vi "rmad mesh to file.vi"(0 "Mote Status":T1(array[cluster]) {"mote state" items=["Lost"=0, "Negotiating"=1, "Operational"=4]}, 3 "mesh datadir":string, 5 "Primary link status":T3(array[cluster]), 9 "last packet type dust":i32[](array[numeric]), 11 "error in":errorcluster, 13 "mac adresses":T2) -> (15 "error out":errorcluster)   [LabVIEW 2017]
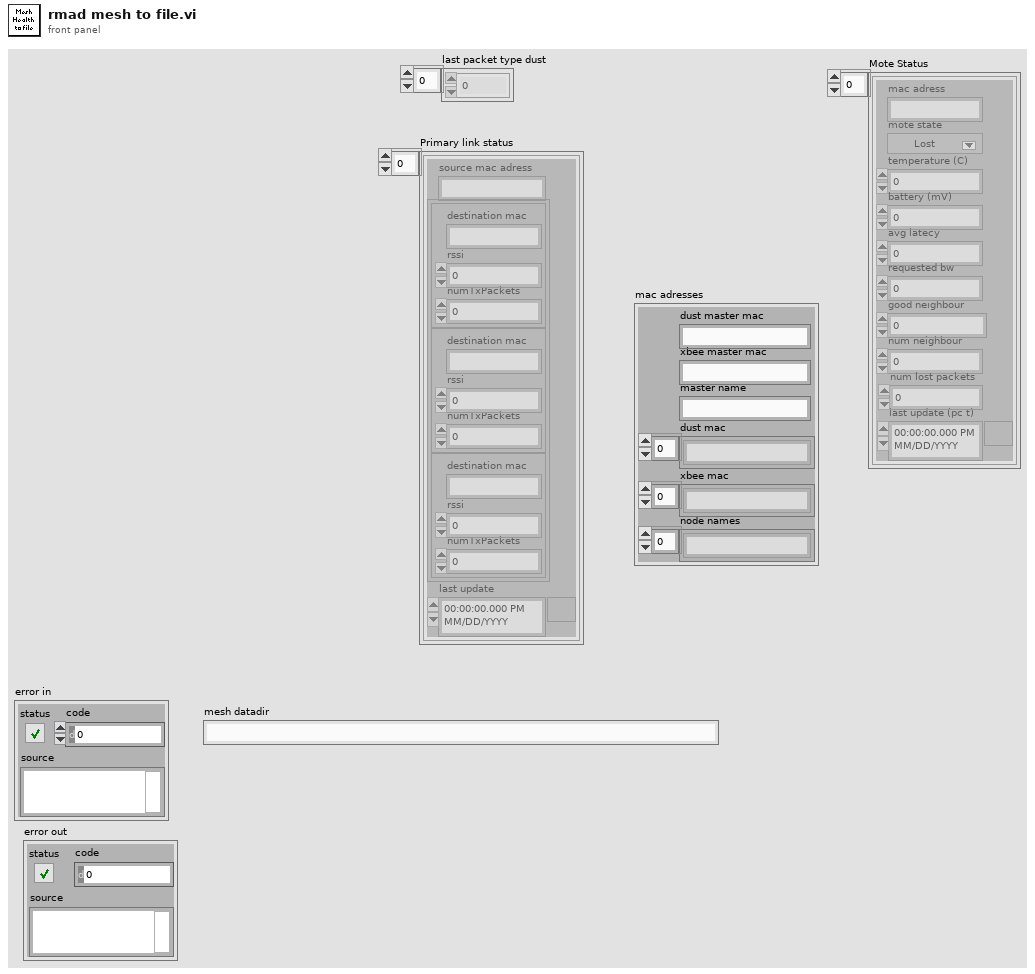
[diagram p1: front panel]
types:
  T1 = cluster{"mac adress":string, "mote state":u8, "temperature (C)":i8, "battery (mV)":u16, "avg latecy":u32, "requested bw":u32, "good neighbour":u8, "num neighbour":u8, "num lost packets":u8, "last update (pc t)":timestamp}[]
  T2 = cluster{"dust master mac":string, "xbee master mac":string, "master name":string, "dust mac":string[], "xbee mac":string[], "node names":string[]}
  T3 = cluster{"source mac adress":string, cluster{"destination mac":string, "rssi":i8, "numTxPackets":u16}[], "last update":timestamp}[]
  T4 = enum16{"open", "replace", "create", "open or create", "replace or create", "replace or create with confirmation"}
  T5 = cluster{"destination mac":string, "rssi":i8, "numTxPackets":u16}[]
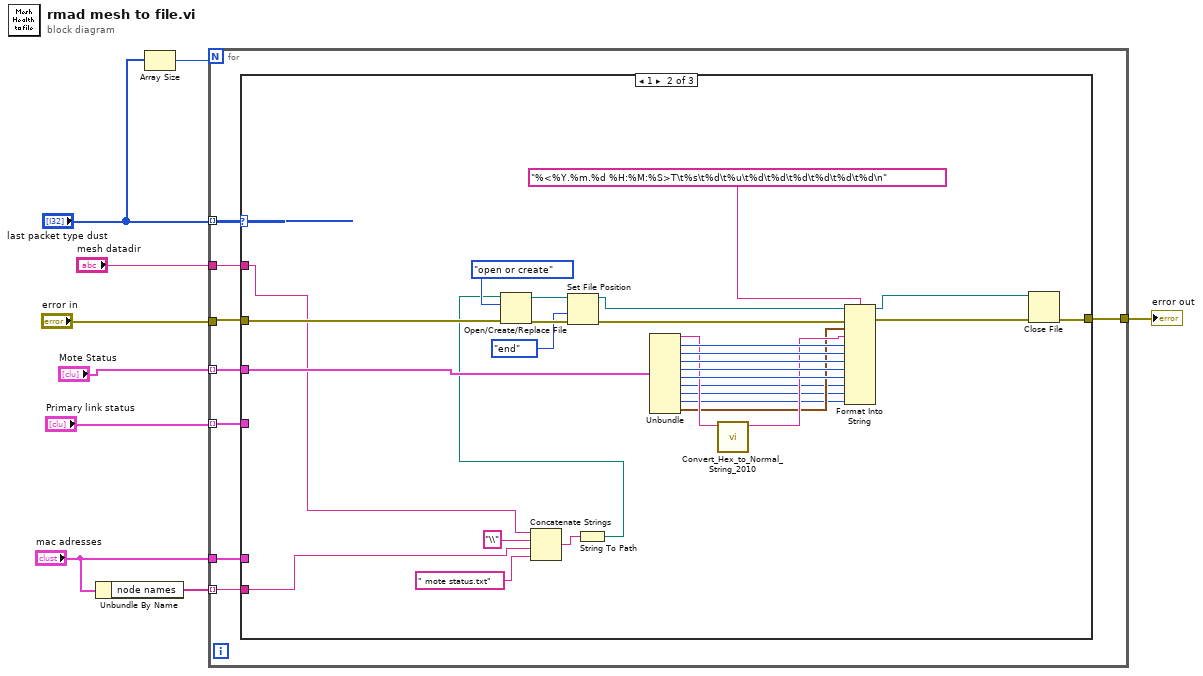
[diagram p0: block diagram]
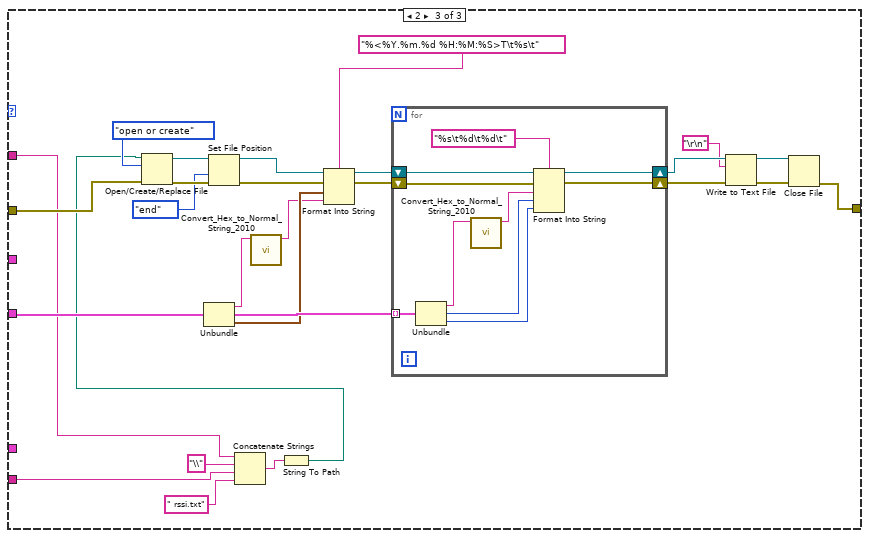
[diagram p3: hidden frame]
diagram:
  n1 = Unbundle By Name("mac adresses") -> ("node names"=w2:string[])
  n2 = Array Size(array="last packet type dust") -> (size(s)=w5:i32)
  n3 = for {
    N: w5 -> [_]
    tunnel: "last packet type dust" -> [w17] mode=indexing
    tunnel: "Mote Status" -> [w16] mode=indexing
    tunnel: "Primary link status" -> [w15] mode=indexing
    tunnel: "error in" -> [w14]
    tunnel: [w13] -> w7
    tunnel: "mesh datadir" -> [w12]
    tunnel: "mac adresses" -> [w11]
    tunnel: w2 -> [w10] mode=indexing
    n4 = case shown="1" w17 {
      tunnel: w16 -> [_ w47 _]
      tunnel: w15 -> [_ _ w74]
      tunnel: w14 -> [w18 w41 w68]
      tunnel: [w18 w40 w67] -> w13
      tunnel: w12 -> [_ w23 w50]
      tunnel: w11 -> [_ _ _]
      tunnel: w10 -> [_ w26 w49]
      frame 0, Default {
      }
      frame 1 {
        n5 = Concatenate Strings(w23, "\\" ("string"), w26, " mote status.txt" ("string")) -> (w28:string)
        n6 = String To Path(string=w28) -> (path=w25:path)
        n7 = Open/Create/Replace File(file path (use dialog)=w25, error in=w41, operation (0:open)=T4."open or create") -> (refnum out=w32:refnum<file>, error out=w34:errorcluster)  [unwired: 3 in, 1 out]
        n8 = Set File Position(refnum=w32, from (0:start)=enum16{"start", "end", "current"}."end", error in=w34) -> (refnum out=w31:refnum<file>, error out=w33:errorcluster)  [unwired: 1 in]
        n9 = Unbundle(w47) -> ("mac adress"=w35:string, "mote state"=w46:u8, "temperature (C)"=w45:i8, "battery (mV)"=w44:u16, "avg latecy"=w43:u32, "requested bw"=w42:u32, "good neighbour"=w21:u8, "num neighbour"=w20:u8, "num lost packets"=w19:u8, "last update (pc t)"=w22:timestamp)
        n10 = call "Convert_Hex_to_Normal_String_2010.vi"("Initial Hex String"=w35) -> ("Normal String - Format into String Method"=w36:string)  [unwired: 8 in]
        n11 = Format Into String(format string="%<%Y.%m.%d %H:%M:%S>T\t%s\t%d\t%u\t%d\t%d\t%d\t%d\t%d\t%d\n", initial string=w31, error in=w33, w22, w36, w46, w45, w44, w43, w42, w21, w20, w19) -> (resulting string=w37:refnum<file>, error out=w39:errorcluster)
        n12 = Close File(refnum=w37, error in=w39) -> (error out=w40:errorcluster)  [unwired: 1 out]
      }
      frame 2 {
        n13 = Unbundle(w74) -> ("source mac adress"=w65:string, w73:T5, "last update"=w66:timestamp)
        n14 = Concatenate Strings(w50, "\\" ("string"), w49, " rssi.txt" ("string")) -> (w52:string)
        n15 = call "Convert_Hex_to_Normal_String_2010.vi"("Initial Hex String"=w65) -> ("Normal String - Format into String Method"=w64:string)  [unwired: 8 in]
        n16 = String To Path(string=w52) -> (path=w51:path)
        n17 = Open/Create/Replace File(file path (use dialog)=w51, error in=w68, operation (0:open)=T4."open or create") -> (refnum out=w70:refnum<file>, error out=w71:errorcluster)  [unwired: 3 in, 1 out]
        n18 = Set File Position(refnum=w70, from (0:start)=enum16{"start", "end", "current"}."end", error in=w71) -> (refnum out=w62:refnum<file>, error out=w63:errorcluster)  [unwired: 1 in]
        n19 = Format Into String(format string="%<%Y.%m.%d %H:%M:%S>T\t%s\t", initial string=w62, error in=w63, w66, w64) -> (resulting string=w61:refnum<file>, error out=w60:errorcluster)
        n20 = for {
          tunnel: w73 -> [w84] mode=indexing
          shift-right: [w79] -> w57
          shift-left: w61 -> [w80]
          shift-right: [w77] -> w58
          shift-left: w60 -> [w78]
          n21 = Unbundle(w84) -> ("destination mac"=w83:string, "rssi"=w81:i8, "numTxPackets"=w75:u16)
          n22 = call "Convert_Hex_to_Normal_String_2010.vi"("Initial Hex String"=w83) -> ("Normal String - Format into String Method"=w82:string)  [unwired: 8 in]
          n23 = Format Into String(format string="%s\t%d\t%d\t", initial string=w80, error in=w78, w82, w81, w75) -> (resulting string=w79:refnum<file>, error out=w77:errorcluster)
        }
        n24 = Write to Text File(file (use dialog)=w57, text="\r\n", error in=w58) -> (refnum out=w56:refnum<file>, error out=w59:errorcluster)  [unwired: 1 in, 1 out]
        n25 = Close File(refnum=w56, error in=w59) -> (error out=w67:errorcluster)  [unwired: 1 out]
      }
    }
  }
  "error out" <- w7
